vi "Shutdown.vi"(8 "error in (no error)":errorcluster, 11 "GE Reflective Memory Transceiver in":refnum<class "GE Reflective Memory Transceiver.lvclass">) -> (0 "error out":errorcluster, 3 "GE Reflective Memory Transceiver out":refnum<class "GE Reflective Memory Transceiver.lvclass">)   [LabVIEW 2017, in "GE Reflective Memory Transceiver.lvlib" / "GE Reflective Memory Transceiver.lvclass"]
uses:
  GE Reflective Memory Transceiver.lvclass
  GE Reflective Memory Transceiver.lvclass/GE Reflective Memory Transceiver.ctl
  <vilib>/NI/GE Reflective Memory Driver/GE 5565PIORC.lvclass
  Transfer Group Parameters.ctl
  <vilib>/NI/GE Reflective Memory Driver/Typedefs/GE 5565PIORC.Typedef.DMA Transfer Spec.ctl
  <vilib>/NI/GE Reflective Memory Driver/Typedefs/GE 5565PIORC.Typedef.DMA Block Descriptor.ctl
  <vilib>/NI/GE Reflective Memory Driver/Typedefs/GE 5565PIORC.Typedef.DMA Block Descriptor Params.ctl
  <vilib>/NI/GE Reflective Memory Driver/GE 5565PIORC.lvclass/GE 5565PIORC.ctl
  <vilib>/NI/GE Reflective Memory Driver/Methods/GE 5565PIORC.DMA.Get Transfer Components (Block).vi
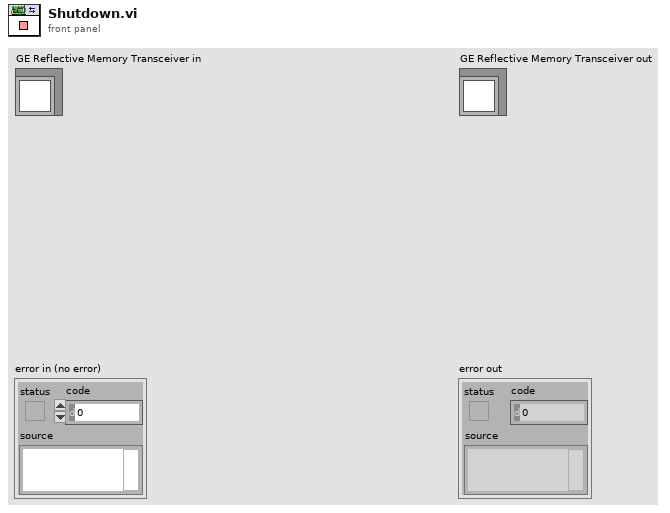
[diagram p1: front panel]
types:
  T1 = typedef "GE Reflective Memory Transceiver.lvlib/GE Reflective Memory Transceiver.lvclass/Transfer Group Parameters.ctl" = cluster{"DMA Transfer Specs":T2[]}
  T2 = typedef "GE 5565PIORC.lvclass/GE 5565PIORC.Typedef.DMA Transfer Spec.ctl" = cluster{"RFM offset":u32, "Block Descriptors":T3[]}
  T3 = typedef "GE 5565PIORC.lvclass/GE 5565PIORC.Typedef.DMA Block Descriptor.ctl" = cluster{"descriptor ptr (VISA)":u32, "descriptor ptr (RFM)":u32, "descriptor size":u32, "descriptor params":T4}
  T4 = typedef "GE 5565PIORC.lvclass/GE 5565PIORC.Typedef.DMA Block Descriptor Params.ctl" = cluster{"data ptr (lower)":u32, "data ptr (upper)":u32, "data size":u32, "next descriptor ptr":u32}
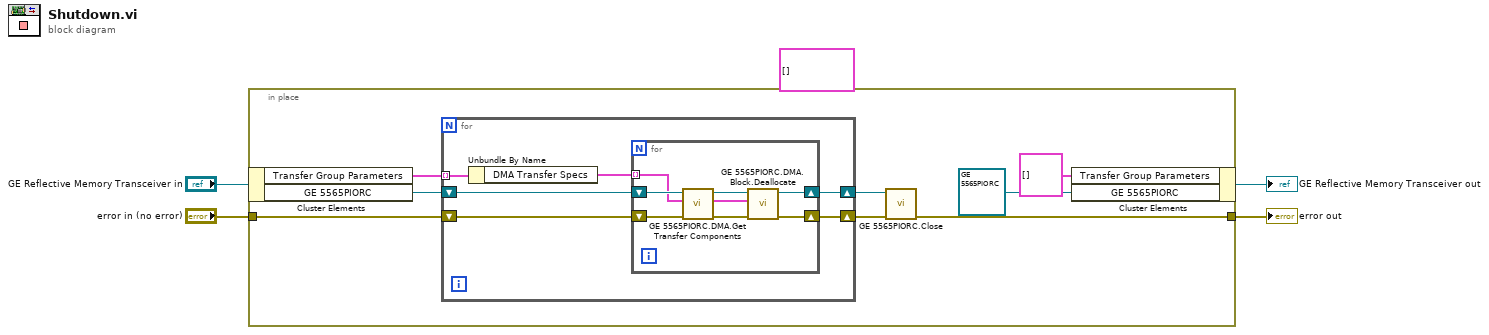
[diagram p0: block diagram]
diagram:
  n1 = in-place {
    in-place-border: "error in (no error)" -> [w10]
    in-place-border: [w9] -> w3
    (unwired) T1[] [] ("Transfer Group Parameters")
    n2 = in-place-cluster #1("GE Reflective Memory Transceiver in") -> ("Transfer Group Parameters"=w7:T1[], "GE 5565PIORC"=w8:refnum<class "GE 5565PIORC.lvclass">)
    n3 = for {
      tunnel: w7 -> [w18] mode=indexing
      shift-right: [w14] -> w12
      shift-left: w10 -> [w16]
      shift-right: [w13] -> w11
      shift-left: w8 -> [w15]
      n4 = Unbundle By Name(w18) -> ("DMA Transfer Specs"=w17:T2[])
      n5 = for {
        tunnel: w17 -> [w24] mode=indexing
        shift-right: [w21] -> w13
        shift-left: w15 -> [w25]
        shift-right: [w19] -> w14
        shift-left: w16 -> [w26]
        n6 = call-poly <vilib>:"GE 5565PIORC.DMA.Get Transfer Components.vi"("error in (no error)"=w26, "DMA Transfer Spec in"=w24, "GE 5565PIORC in"=w25) -> ("error out"=w20:errorcluster, "Block Descriptor"=w23:T3, "GE 5565PIORC out"=w22:refnum<class "GE 5565PIORC.lvclass">)  [unwired: 5 in, 1 out]
        n7 = call <vilib>:"GE 5565PIORC.DMA.Block.Deallocate.vi"("error in (no error)"=w20, "Block Descriptor"=w23, "GE 5565PIORC in"=w22) -> ("error out"=w19:errorcluster, "GE 5565PIORC out"=w21:refnum<class "GE 5565PIORC.lvclass">)  [unwired: 7 in]
      }
    }
    n8 = call <vilib>:"GE 5565PIORC.Close.vi"("error in (no error)"=w12, "GE 5565PIORC in"=w11) -> ("error out"=w9:errorcluster)  [unwired: 8 in, 1 out]
    n9 = in-place-cluster #1("Transfer Group Parameters"=T1[] [], "GE 5565PIORC"=refnum<class "GE 5565PIORC.lvclass"> refnum) -> (→"GE Reflective Memory Transceiver out":refnum<class "GE Reflective Memory Transceiver.lvclass">)
  }
  "error out" <- w3
